vi "CANOpen_Main_Close xPDOs.vi"(8 "error in (no error)":errorcluster, 11 "xPDO Refs":T1) -> (0 "error out":errorcluster)   [LabVIEW 2021, in "CANOpen Addon Engine.lvlib"]
uses:
  CANOpen Addon Engine.lvlib
  CANOpen_xPDO Refs.ctl
  CanOpen_RPDO Refs.ctl
  CanOpen_TPDO Refs.ctl
  <vilib>/CANopenLib/CANOPEN.llb/CANopen RPDO Close.vi
  <vilib>/CANopenLib/CANOPEN.llb/CANopen TPDO Close.vi
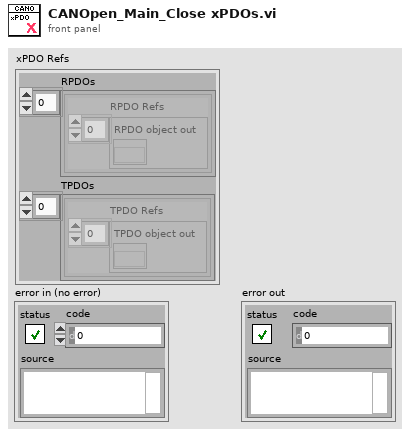
[diagram p1: front panel]
types:
  T1 = typedef "CANOpen Addon Engine.lvlib/CANOpen_xPDO Refs.ctl" = cluster{"RPDOs":T2[], "TPDOs":T3[]}
  T2 = typedef "CANOpen Addon Engine.lvlib/CanOpen_RPDO Refs.ctl" = cluster{"RPDO Refs":refnum<k20>[]}
  T3 = typedef "CANOpen Addon Engine.lvlib/CanOpen_TPDO Refs.ctl" = cluster{"TPDO Refs":refnum<k20>[]}
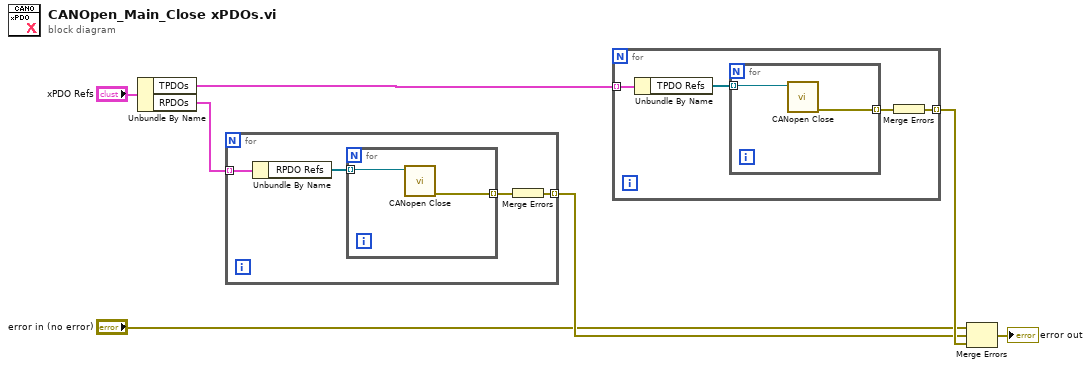
[diagram p0: block diagram]
diagram:
  n1 = Unbundle By Name("xPDO Refs") -> ("TPDOs"=w1:T3[], "RPDOs"=w7:T2[])
  n2 = for {
    tunnel: w7 -> [w11] mode=indexing
    tunnel: [w8] -> w4 mode=indexing
    n3 = Unbundle By Name(w11) -> ("RPDO Refs"=w10:refnum<k20>[])
    n4 = for {
      tunnel: w10 -> [w13] mode=indexing
      tunnel: [w12] -> w9 mode=indexing
      n5 = call-poly <vilib>:"CANopen Close.vi"("RPDO object in"=w13) -> ("error out"=w12:errorcluster)  [unwired: 10 in]
    }
    n6 = Merge Errors(w9) -> (w8:errorcluster)
  }
  n7 = for {
    tunnel: w1 -> [w17] mode=indexing
    tunnel: [w14] -> w5 mode=indexing
    n8 = Unbundle By Name(w17) -> ("TPDO Refs"=w16:refnum<k20>[])
    n9 = for {
      tunnel: w16 -> [w19] mode=indexing
      tunnel: [w18] -> w15 mode=indexing
      n10 = call-poly <vilib>:"CANopen Close.vi"("TPDO object in"=w19) -> ("error out"=w18:errorcluster)  [unwired: 10 in]
    }
    n11 = Merge Errors(w15) -> (w14:errorcluster)
  }
  n12 = Merge Errors("error in (no error)", w4, w5) -> (→"error out":errorcluster)
